vi "Find Complete Frame.vi"(8 "error in (no error)":errorcluster, 10 "Read Buffer in":string, 11 "iTacho in":refnum<class "iTacho.lvclass">) -> (0 "error out":errorcluster, 1 "Found New Frame?":bool, 2 "Frame":string, 3 "iTacho out":refnum<class "iTacho.lvclass">, 4 "Left Over Bytes":string)   [LabVIEW 2017, in "iTacho.lvclass"]
uses:
  iTacho.lvclass
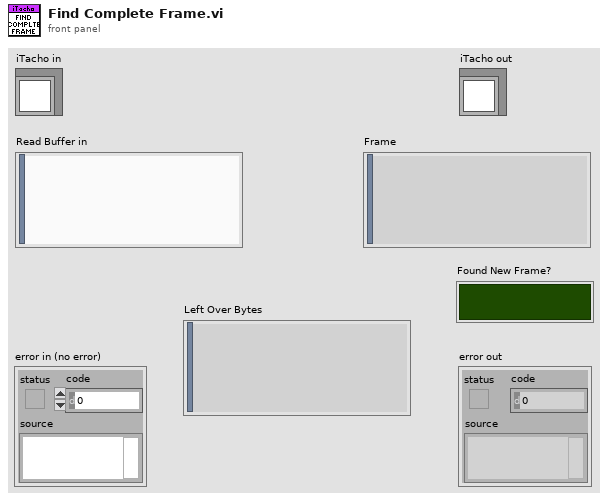
[diagram p1: front panel]
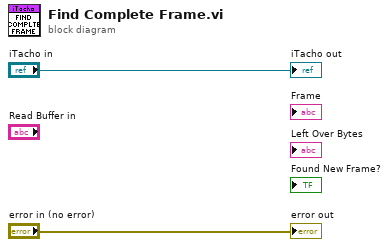
[diagram p0: block diagram]
diagram:
  "error out" <- "error in (no error)"
  "iTacho out" <- "iTacho in"
